vi "GetHostTime.vi"() -> (0 "current time":timestamp)   [LabVIEW 2012]
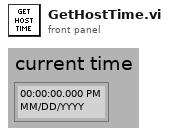
[diagram p1: front panel]
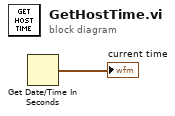
[diagram p0: block diagram]
diagram:
  n1 = Get Date/Time In Seconds() -> (seconds since 1Jan1904=→"current time":timestamp)
